vi "USBCLIENT1.vi"() -> ()   [LabVIEW 2018]
uses:
  <vilib>/daq.io/MQTT LabVIEW Client/Controls/QoS.ctl
  <vilib>/daq.io/MQTT LabVIEW Client/Controls/DUP_Flag.ctl
  <vilib>/daq.io/MQTT LabVIEW Client/Controls/Retain_Flag.ctl
  <vilib>/daq.io/MQTT LabVIEW Client/Controls/Connect_Flags.ctl
  <vilib>/daq.io/MQTT LabVIEW Client/Controls/User_Info.ctl
  <vilib>/DAQmx/read.llb/DAQmx Read (Analog DBL 1Chan 1Samp).vi
  <vilib>/DAQmx/write.llb/DAQmx Write (Digital Bool 1Line 1Point).vi
  <vilib>/DAQmx/create/channels.llb/DAQmx Create Channel (AI-Voltage-Basic).vi
  <vilib>/DAQmx/create/channels.llb/DAQmx Create Channel (DO-Digital Output).vi
  <vilib>/DAQmx/miscellaneous.llb/DAQmx Fill In Error Info.vi
  <vilib>/daq.io/MQTT LabVIEW Client/MQTT_Functions.lvlib
panel:
  in  "stop":bool
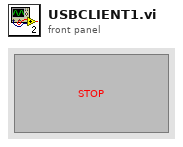
[diagram p1: front panel]
types:
  T1 = typedef "MQTT_Functions.lvlib/User_Info.ctl" = cluster{"User Name":string, "Password":string}
  T2 = typedef "MQTT_Functions.lvlib/QoS.ctl" = enum8{"At most once", "At least once", "Exactly once", "Reserved"}
  T3 = typedef "MQTT_Functions.lvlib/Connect_Flags.ctl" = cluster{"user name":bool, "password":bool, "will retain":bool, "will flag":bool, "clean session":bool, "reserved":bool, "will QoS":T2}
  T4 = typedef "MQTT_Functions.lvlib/DUP_Flag.ctl" = bool
  T5 = typedef "MQTT_Functions.lvlib/Retain_Flag.ctl" = bool
  T6 = cluster{"QoS":T2, "DUP":T4, "Retain":T5, "Keep Alive (sec)":u16}
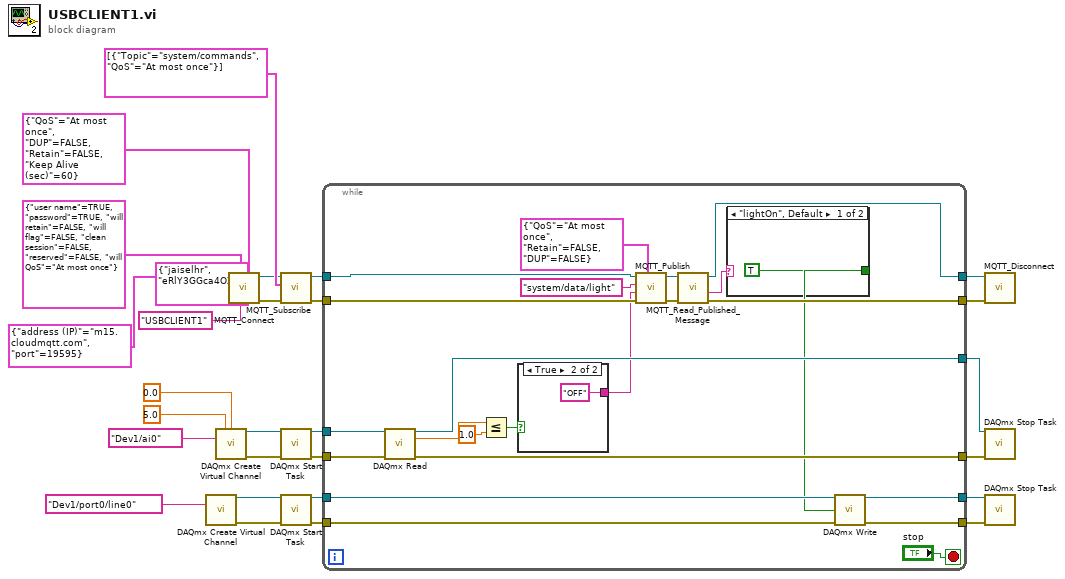
[diagram p0: block diagram]
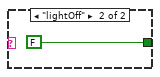
[diagram p2: hidden frame]
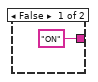
[diagram p3: hidden frame]
diagram:
  n1 = call-poly <vilib>:"DAQmx Create Virtual Channel.vi"("lines"=tag "Dev1/port0/line0") -> ("task out"=w7:refnum<k21>, "error out"=w6:errorcluster)  [unwired: 13 in]
  n2 = call-poly <vilib>:"DAQmx Create Virtual Channel.vi"("maximum value"=5.0, "minimum value"=0.0, "physical channels"=tag "Dev1/ai0") -> ("task out"=w16:refnum<k21>, "error out"=w15:errorcluster)  [unwired: 11 in]
  n3 = call <vilib>:"MQTT_Connect.vi"("Connect Meta"=T6 {"QoS"=enum."At most once", "DUP"=FALSE, "Retain"=FALSE, "Keep Alive (sec)"=60}, "Client ID"="USBCLIENT1", "Connect Flags"=T3 {"user name"=TRUE, "password"=TRUE, "will retain"=FALSE, "will flag"=FALSE, "clean session"=FALSE, "reserved"=FALSE, "will QoS"=enum."At most once"}, "User Info"=T1 {"User Name"="jaiselhr", "Password"="eRlY3GGca4OZ"}, "MQTT Broker"=cluster{"address (IP)":string, "port":u16} {"address (IP)"="m15.cloudmqtt.com", "port"=19595}) -> ("error out"=w22:errorcluster, "connection ID out"=w20:refnum<k5>)  [unwired: 4 in, 1 out]
  n4 = call <vilib>:"MQTT_Subscribe.vi"("error in (no error)"=w22, "Subscription Info Array"=cluster{"Topic":string, "QoS":T2}[] [{"Topic"="system/commands", "QoS"=enum."At most once"}], "connection ID"=w20) -> ("error out"=w19:errorcluster, "connection ID out"=w18:refnum<k5>)  [unwired: 7 in]
  n5 = call <vilib>:"DAQmx Start Task.vi"("task/channels in"=w16, "error in"=w15) -> ("task out"=w12:refnum<k21>, "error out"=w11:errorcluster)  [unwired: 12 in]
  n6 = call <vilib>:"DAQmx Start Task.vi"("task/channels in"=w7, "error in"=w6) -> ("task out"=w5:refnum<k21>, "error out"=w4:errorcluster)  [unwired: 12 in]
  n7 = while {
    tunnel: [w49] -> w24
    tunnel: [w48] -> w23
    tunnel: w19 -> [w47]
    tunnel: w18 -> [w46]
    tunnel: w12 -> [w44]
    tunnel: w11 -> [w43]
    tunnel: [w42] -> w10
    tunnel: [w41] -> w9
    tunnel: w5 -> [w33]
    tunnel: w4 -> [w32]
    tunnel: [w30] -> w3
    tunnel: [w29] -> w2
    stop <- "stop" stop-if-true
    n8 = call-poly <vilib>:"DAQmx Read.vi"("task/channels in"=w44, "error in"=w43) -> ("task out"=w42:refnum<k21>, "data"=w39:dbl, "error out"=w41:errorcluster)  [unwired: 11 in]
    n9 = Less Or Equal?(x=w39, y=1.0) -> (x <= y?=w37:bool)
    n10 = case shown="True" w37 {
      tunnel: ["ON" ("Message to be published") "OFF" ("Message to be published")] -> w36
      frame False {
      }
      frame True {
      }
    }
    n11 = call <vilib>:"MQTT_Publish.vi"("Publish Meta"=cluster{"QoS":T2, "Retain":T5, "DUP":T4} {"QoS"=enum."At most once", "Retain"=FALSE, "DUP"=FALSE}, "error in (no error)"=w47, "Message to be published"=w36, "Topic"="system/data/light", "connection ID"=w46) -> ("error out"=w51:errorcluster, "connection ID out"=w50:refnum<k5>)  [unwired: 5 in]
    n12 = call <vilib>:"MQTT_Read_Published_Message.vi"("error in (no error)"=w51, "connection ID"=w50) -> ("error out"=w49:errorcluster, "Message"=w34:string, "connection ID out"=w48:refnum<k5>)  [unwired: 4 in, 3 out]
    n13 = case shown="\"lightOn\", Default" w34 {
      tunnel: [TRUE ("data") FALSE ("data")] -> w31
      frame "lightOn", Default {
      }
      frame "lightOff" {
      }
    }
    n14 = call-poly <vilib>:"DAQmx Write.vi"("task/channels in"=w33, "data"=w31, "error in"=w32) -> ("task out"=w30:refnum<k21>, "error out"=w29:errorcluster)  [unwired: 10 in, 1 out]
  }
  n15 = call <vilib>:"MQTT_Disconnect.vi"("error in (no error)"=w24, "connection ID"=w23) -> ()  [unwired: 9 in, 1 out]
  n16 = call <vilib>:"DAQmx Stop Task.vi"("task/channels in"=w10, "error in"=w9) -> ()  [unwired: 12 in, 2 out]
  n17 = call <vilib>:"DAQmx Stop Task.vi"("task/channels in"=w3, "error in"=w2) -> ()  [unwired: 12 in, 2 out]
